vi "read XYZ piezos property names.vi"(5 "error in (no error)":errorcluster) -> (14 "XYZ piezos":string[](array[string]), 19 "error out":errorcluster)   [LabVIEW 2019, in "metadata.lvclass"]
uses:
  metadata.lvclass
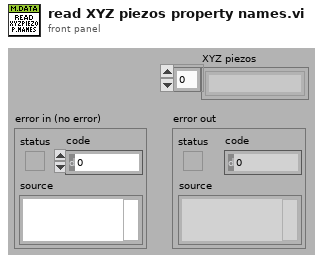
[diagram p1: front panel]
types:
  T1 = typedef "metadata.lvclass/ClassAttributesRef.ctl" = refnum<data-value>
  T2 = typedef "metadata.lvclass/ClassAttributes.ctl" = cluster{"File":bool, "Cantilever":bool, "System control":bool, "XYZ piezos":bool, "Sample info":bool, "Fast fpga param":bool, "Mapping param":bool, "Chirp param":bool, "Fcurve Seg":bool, "Property names":cluster{"File info":string[], "Cantilever calib":string[], "System control":string[], "XYZ piezos":string[], "Sample info":string[], "Fast fpga param":string[], "Mapping param":string[], "Chirp Param":string[], "Fcurve Seg":string[]}}
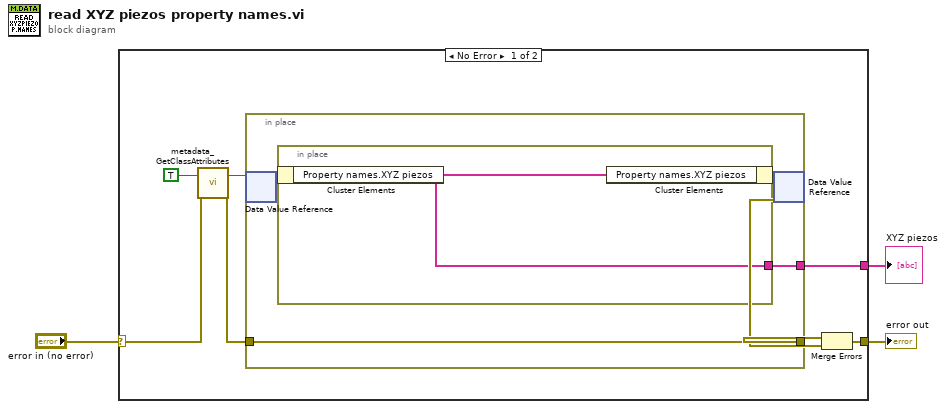
[diagram p0: block diagram]
diagram:
  n1 = case shown="No Error" "error in (no error)" {
    selector: "error in (no error)" -> [w11 w17]
    tunnel: [w8 w17] -> w2
    tunnel: [w4 _] -> w1
    frame No Error {
      n2 = call "metadata_GetClassAttributes.vi"("return data? (T)"=TRUE ("return data"), "error in (no error)"=w11) -> ("class attributes ref"=w9:T1, "error out"=w10:errorcluster)  [unwired: 14 in, 2 out]
      n3 = in-place {
        in-place-border: w10 -> [w13]
        in-place-border: [w13] -> w6
        in-place-border: [w12] -> w4
        n4 = in-place-dvr #1(w9) -> (w14:T2)  [unwired: 1 out]
        n5 = in-place {
          in-place-border: [w16] -> w12
          n6 = in-place-cluster #2(w14) -> ("Property names.XYZ piezos"=w16:string[])
          n7 = in-place-cluster #2("Property names.XYZ piezos"=w16) -> (w15:T2)
        }
        n8 = in-place-dvr #1(w15) -> (w5:errorcluster)  [unwired: 1 out]
      }
      n9 = Merge Errors(w6, w5) -> (w8:errorcluster)
    }
    frame Error {
    }
  }
  "error out" <- w2
  "XYZ piezos" <- w1
